vi "PS_TestCOM.vi"() -> ()   [LabVIEW 2012]
uses:
  SubVIs/LVPresent_Globals.vi
  <userlib>/BotSpeak/VIs/SubVIs/BotSpeak_Globals.vi
  BotSpeakSubs/BotspeakSettingsUsed.vi
panel:
  out "Status":string
  out "List":string[](array[string])
  in  "Test Button":bool
  in  "Com Port":u16(ring)
  in  "Hardware":u16(ring) items=["Arduino Uno", "BeagleBone Serial", "BeagleBone", "Console Only", "EV3", "EvalRIO", "Launchpad", "PICAXE 80M", "Raspberry Pi", "Thymio"]
  out "Connect?":bool
  # "Test BotSpeak\n\nThe next step is to test it out.  Choose your hardware and port (if you have not plugged your Protosnap in yet, plug it in and select Arduino Uno). You should get a green square after a few seconds if you are connected. Click the next arrow once you are connected."
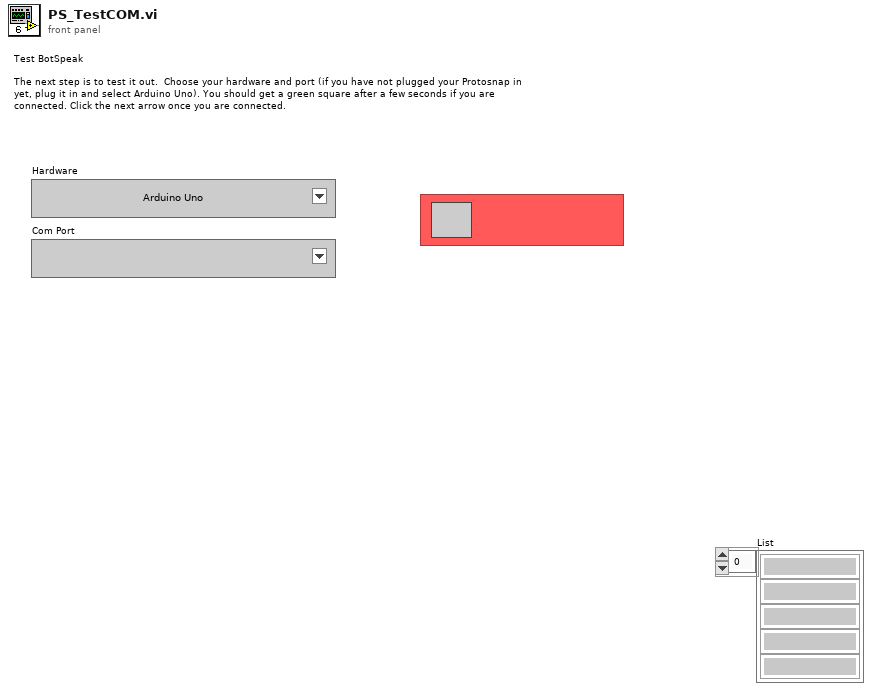
[diagram p1: front panel]
types:
  T1 = typedef "BotSpeak.HardwareSpecs.ctl" = cluster{"Hardware Name":string, "Hardware URL":string, "ComType":enum16{"Undefined", "Serial", "TCPIP", "Console", "EV3"}, "TCP Port":i32, "DefaultAddress":string, "Retries":i32, "Translate":enum16{"None", "Tiny", "URAPI"}, "MaxScriptSize":i32, "MaxVarNumber":i32, "StartupWait":i32, "Patience":i32, "Startup Patience":i32, "Hardware Help":string, "Com Protocol":string, "Translator":cluster{"BotSpeak CMD":string, "CMD out":string}[], "Init Code":string, "Variable Format":enum16{"INT", "FLOAT", "FIXED"}}
  T2 = enum16{"Undefined", "Serial", "TCPIP", "Console", "EV3"}
  T3 = typedef "BotSpeak_Control.ctl" = cluster{"Address":string, "Reply EOF":string, "Hardware":string, "Retries":i8, "Timeout":i32}
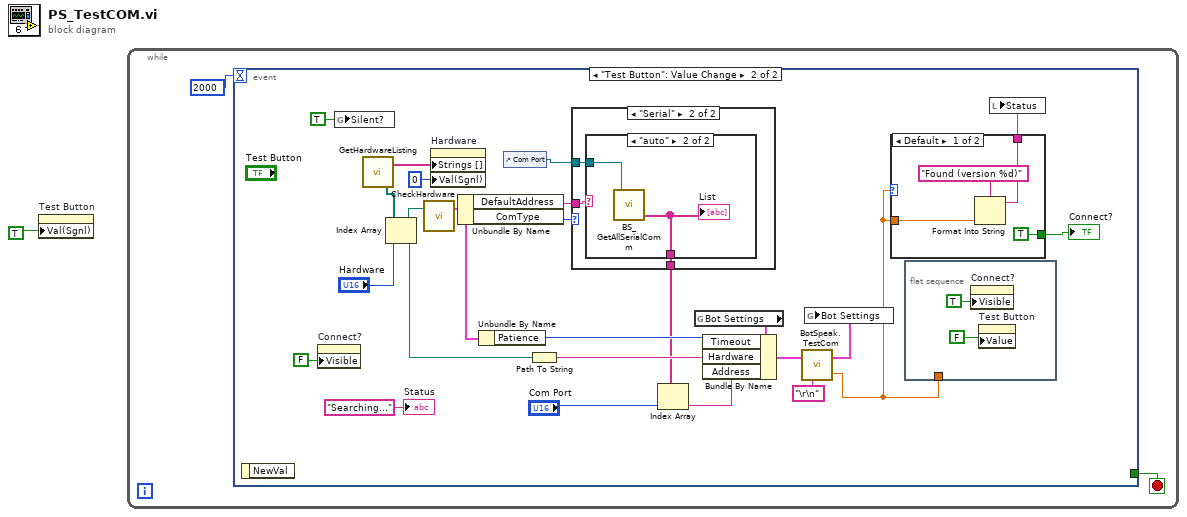
[diagram p0: block diagram]
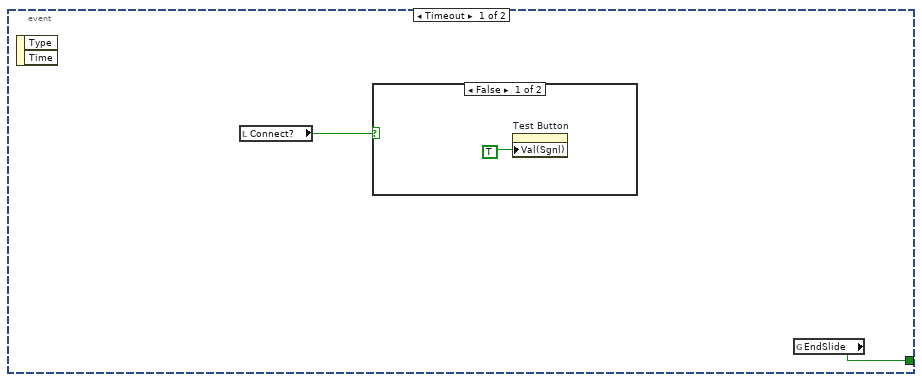
[diagram p2: hidden frame]
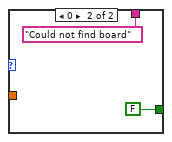
[diagram p4: hidden frame]
diagram:
  n1 = property on="Test Button" class="Bool (strict)"("Val(Sgnl)"=TRUE) -> ()  [unwired: 2 in, 2 out]
  n2 = while {
    stop <- w3 stop-if-true
    n3 = event shown="[1] \"Test Button\": Value Change" {
      selector: _ -> [_ _]
      dyn-events: _ -> [_ _]
      timeout: 2000 -> [_ _]
      tunnel: [w5 _] -> w3
      event Timeout {
        n4 = event-data() -> ()  [unwired: 1 in, 2 out]
        n5 = local read "Connect?"() -> (w4:bool)
        n6 = case shown="False" w4 {
          frame False {
            n7 = property on="Test Button" class="Bool (strict)"("Val(Sgnl)"=TRUE) -> ()  [unwired: 2 in, 2 out]
          }
          frame True {
          }
        }
        n8 = global read "LVPresent_Globals.vi" "EndSlide"() -> (w5:bool)
      }
      event "Test Button": Value Change {
        n9 = event-data() -> ()  [unwired: 1 in, 1 out]
        n10 = property on="Connect?" class="Bool (strict)"("Visible"=FALSE) -> ()  [unwired: 2 in, 2 out]
        n11 = global write "BotSpeak_Globals.vi" "Silent?"(TRUE ("Silent?")) -> ()
        n12 = call <userlib>:"GetHardwareListing.vi"() -> ("Devices"=w19:path[], "Array"=w26:string[])  [unwired: 2 in]
        n13 = Index Array(array=w19, index="Hardware") -> (element=w18:path)
        n14 = call <userlib>:"CheckHardware.vi"("Hardware"=w18) -> ("HardwareSpecs"=w14:T1)  [unwired: 2 in]
        n15 = property on="Hardware" class="Ring (strict)"("Strings []"=w26, "Val(Sgnl)"=u16 0 ("Value (Signaling)")) -> ()  [unwired: 2 in, 2 out]
        n16 = Unbundle By Name(w14) -> ("DefaultAddress"=w28:string, "ComType"=w29:T2)
        n17 = Unbundle By Name(w14) -> ("Patience"=w23:i32)
        n18 = control-ref of="Com Port"() -> (w30:refnum<vi>)
        n19 = Path To String(path=w18) -> (string=w24:string)
        n20 = case shown="\"Serial\"" w29 {
          tunnel: w28 -> [_ w39]
          tunnel: w30 -> [_ w38]
          tunnel: [_ w37] -> w15
          frame Default {
          }
          frame "Serial" {
            n21 = case shown="\"auto\"" w39 {
              tunnel: w38 -> [_ w41]
              tunnel: [_ w40] -> w37
              frame Default {
              }
              frame "auto" {
                n22 = call <userlib>:"BS_GetAllSerialComm.vi"("reference"=w41) -> ("List"=w40:string[])  [unwired: 1 in, 2 out]
                "List" <- w40
              }
            }
          }
        }
        n23 = Index Array(array=w15, index="Com Port") -> (element=w22:string)
        n24 = global read "BotspeakSettingsUsed.vi" "Bot Settings"() -> (w17:T3)
        n25 = Bundle By Name(cluster=w17, "Timeout"=w23, "Hardware"=w24, "Address"=w22) -> (w21:T3)
        n26 = call <userlib>:"BotSpeak.TestCom.vi"("Termination"="\r\n", "Bot Settings"=w21) -> ("firmware"=w11:dbl, "Bot Settings out"=w13:T3)
        n27 = global write "BotspeakSettingsUsed.vi" "Bot Settings"(w13) -> ()
        n28 = case shown="Default" w11 {
          tunnel: w11 -> [w33 _]
          tunnel: [w32 "Could not find board"] -> w10
          tunnel: [TRUE FALSE] -> w9
          frame Default {
            n29 = Format Into String(format string="Found (version %d)" ("Status"), w33) -> (resulting string=w32:string)  [unwired: 2 in, 1 out]
          }
          frame 0 {
          }
        }
        "Connect?" <- w9
        n30 = flat-sequence {
          tunnel: w11 -> [_]
          frame #0 {
            n31 = property on="Connect?" class="Bool (strict)"("Visible"=TRUE) -> ()  [unwired: 2 in, 2 out]
            n32 = property on="Test Button" class="Bool (strict)"("Value"=FALSE) -> ()  [unwired: 2 in, 2 out]
          }
        }
        n33 = local write "Status"(w10) -> ()
        "Status" <- "Searching..." ("Status")
      }
    }
  }
